vi "Host - Get Local and ECAT Masters.vi"(8 "error in (no error)":errorcluster, 11 "Refnum in":refnum<k21>) -> (0 "error out":errorcluster, 1 "Local UDV Container":refnum<k21>[](array[refnum]), 2 "All Local Mods":refnum<k21>[](array[refnum]), 3 "All ECAT Masters":refnum<k21>[](array[refnum]))   [LabVIEW 2020, in "SEECD System Explorer.lvlib"]
uses:
  SEECD System Explorer.lvlib
  <resource>/objmgr/ni.var.rc
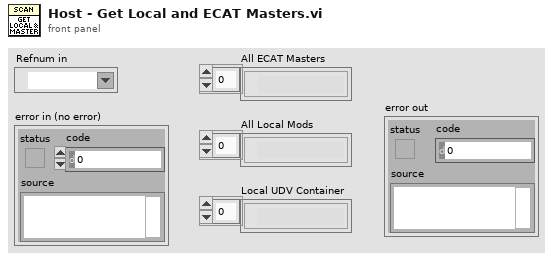
[diagram p1: front panel]
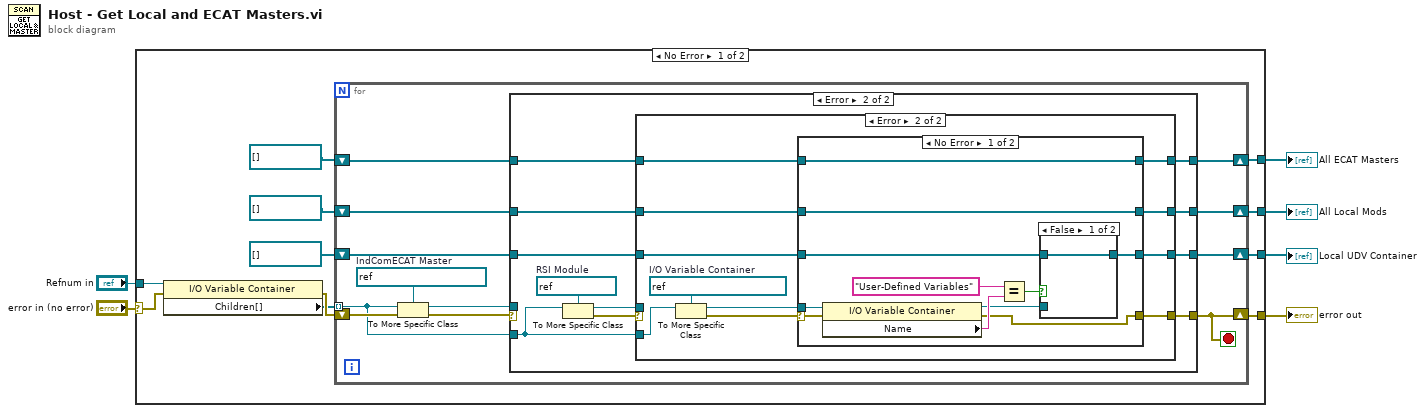
[diagram p0: block diagram]
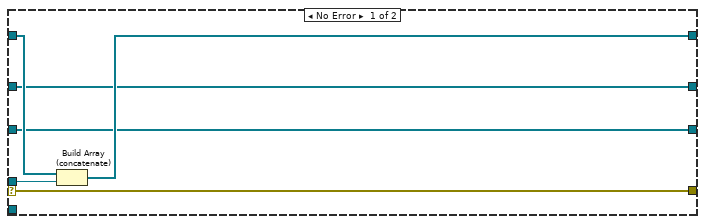
[diagram p2: hidden frame]
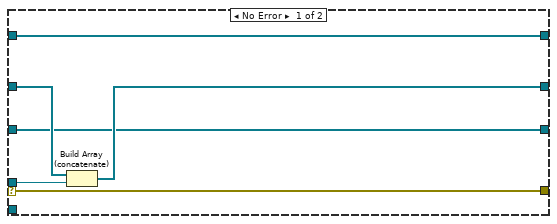
[diagram p3: hidden frame]
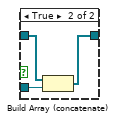
[diagram p4: hidden frame]
diagram:
  n1 = case shown="No Error" "error in (no error)" {
    selector: "error in (no error)" -> [w7 w83]
    tunnel: "Refnum in" -> [w8 _]
    tunnel: [w17 _] -> w5
    tunnel: [w16 _] -> w4
    tunnel: [w15 _] -> w3
    tunnel: [w9 w83] -> w2
    frame No Error {
      n2 = property class="I/O Variable Container"(reference=w8, error in=w7) -> (error out=w14:errorcluster, "Children[]"=w13:refnum<k21>[])  [unwired: 1 out]
      n3 = for {
        tunnel: w13 -> [w23] mode=indexing
        shift-right: [w25] -> w17
        shift-left: refnum<k21>[] [] -> [w24]
        shift-right: [w21] -> w15
        shift-left: refnum<k21>[] [] -> [w22]
        shift-right: [w19] -> w16
        shift-left: refnum<k21>[] [] -> [w20]
        shift-right: [w18] -> w9
        shift-left: w14 -> [w29]
        stop <- w18 stop-if-true
        w28 = refnum<k21> refnum  # IndComECAT Master
        n4 = To More Specific Class(target class=w28, reference=w23, error in=w29) -> (specific class reference=w26:refnum<k21>, error out=w27:errorcluster)
        n5 = case shown="Error" w27 {
          selector: w27 -> [w33 _]
          tunnel: w26 -> [w30 _]
          tunnel: [w35 w40] -> w25
          tunnel: w24 -> [w34 w41]
          tunnel: [w33 w39] -> w18
          tunnel: w23 -> [_ w38]
          tunnel: w22 -> [w32 w43]
          tunnel: [w32 w42] -> w21
          tunnel: w20 -> [w31 w37]
          tunnel: [w31 w36] -> w19
          frame No Error {
            n6 = Build Array (concatenate)(w34, w30) -> (w35:refnum<k21>[])
          }
          frame Error {
            w46 = refnum<k21> refnum  # RSI Module
            n7 = To More Specific Class(target class=w46, reference=w38) -> (specific class reference=w44:refnum<k21>, error out=w45:errorcluster)  [unwired: 1 in]
            n8 = case shown="Error" w45 {
              tunnel: w44 -> [w48 _]
              selector: w45 -> [w47 _]
              tunnel: w43 -> [w52 w59]
              tunnel: [w51 w56] -> w42
              tunnel: w41 -> [w50 w58]
              tunnel: [w50 w57] -> w40
              tunnel: [w47 w53] -> w39
              tunnel: w38 -> [_ w62]
              tunnel: w37 -> [w49 w60]
              tunnel: [w49 w55] -> w36
              frame No Error {
                n9 = Build Array (concatenate)(w52, w48) -> (w51:refnum<k21>[])
              }
              frame Error {
                w63 = refnum<k21> refnum  # I/O Variable Container
                n10 = To More Specific Class(target class=w63, reference=w62) -> (specific class reference=w54:refnum<k21>, error out=w61:errorcluster)  [unwired: 1 in]
                n11 = case shown="No Error" w61 {
                  selector: w61 -> [w72 w79]
                  tunnel: w60 -> [w66 w82]
                  tunnel: w59 -> [w73 w81]
                  tunnel: w58 -> [w74 w80]
                  tunnel: [w74 w80] -> w57
                  tunnel: [w73 w81] -> w56
                  tunnel: [w65 w82] -> w55
                  tunnel: w54 -> [w71 _]
                  tunnel: [w64 w79] -> w53
                  frame No Error {
                    n12 = property class="I/O Variable Container"(reference=w71, error in=w72) -> (reference out=w67:refnum<k21>, error out=w64:errorcluster, "Name"=w70:string)
                    n13 = Equal?(x="User-Defined Variables", y=w70) -> (x = y?=w68:bool)
                    n14 = case shown="False" w68 {
                      tunnel: w67 -> [_ w77]
                      tunnel: w66 -> [w75 w78]
                      tunnel: [w75 w76] -> w65
                      frame False {
                      }
                      frame True {
                        n15 = Build Array (concatenate)(w78, w77) -> (w76:refnum<k21>[])
                      }
                    }
                  }
                  frame Error {
                  }
                }
              }
            }
          }
        }
      }
    }
    frame Error {
    }
  }
  "All ECAT Masters" <- w5
  "Local UDV Container" <- w4
  "All Local Mods" <- w3
  "error out" <- w2
